vi "Project Open.vi"(8 "error in":errorcluster, 11 "File Path":path) -> (0 "error out":errorcluster caption="错误输出")   [LabVIEW 2016]
uses:
  DAQ-VirtualCH/SubVIs/VCH/Private/Ctrls/PSVCH_VCH Info.ctl
  DAQ-Config/SubVIs/FGV_Cards.ctl
  DAQ-Display/Controls/Global para Config.ctl
  DAQ-Config/Controls/PSCHN_Card Para.ctl
  DAQ-Config/Controls/PSCHN_Channel Para.ctl
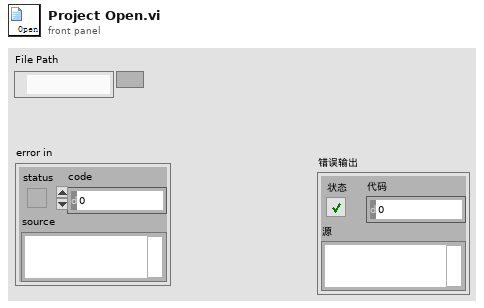
[diagram p1: front panel]
types:
  T1 = typedef "PSVCH_VCH Info.ctl" = cluster{"Tag":string[], "Tag String":string[], "Name":string[], "Enable":bool[], "Formula":string[], "Unit":string[], "Save":bool[], "Time":i64[]}
  T2 = typedef "Global para Config.ctl" = cluster{"连续存储设置":cluster{"Save Mode":i32, "Sel Save Mode":i32, "FolderPath":path, "Filename":string, "Explation":string, "AutoPoint":i32, "Template":path}, "Latest Prj":path, "Tdms Ref*":refnum<k34>, "默认波形图个数":u8, "列表列数":u8}
  T3 = typedef "PSCHN_Card Para.ctl" = cluster{"Module Type":string, "Module Name":string, "ModuSN":string, "ModuIP":string, "Used?":bool, "Connected":bool, "Timing*":cluster{"Sample Rate":dbl}, "Channels":T4[]}
  T4 = typedef "PSCHN_Channel Para.ctl" = cluster{"CHTag*":string, "Used?*":bool, "CHName":string, "Unit":string, "斜率":dbl, "截距":dbl}
  T5 = cluster{"DispXml[]":string[], "VCH Out":T1, "_Para":T2, "Cards":T3[], "CHTag[]":string[]}
  T6 = typedef "FGV_Cards.ctl" = enum16{"Initlize", "Set_DAQCards", "Set_VCHCards", "Get_DAQCards", "Get_VCHCards", "Get_ALLUsing"}
  T7 = enum16{"Run", "Pause", "Stop", "DAQ Chl", "Save", "Update Data", "Symbol Path", "DAQ DATA Queues", "None"}
  T8 = cluster{"Main Queue":string, "DAQ Queue":string, "ANA Queue":string, "CUI Queue":string, "Q-FocusList":string, "Q-Toolbar":string, "Q-Config":string}
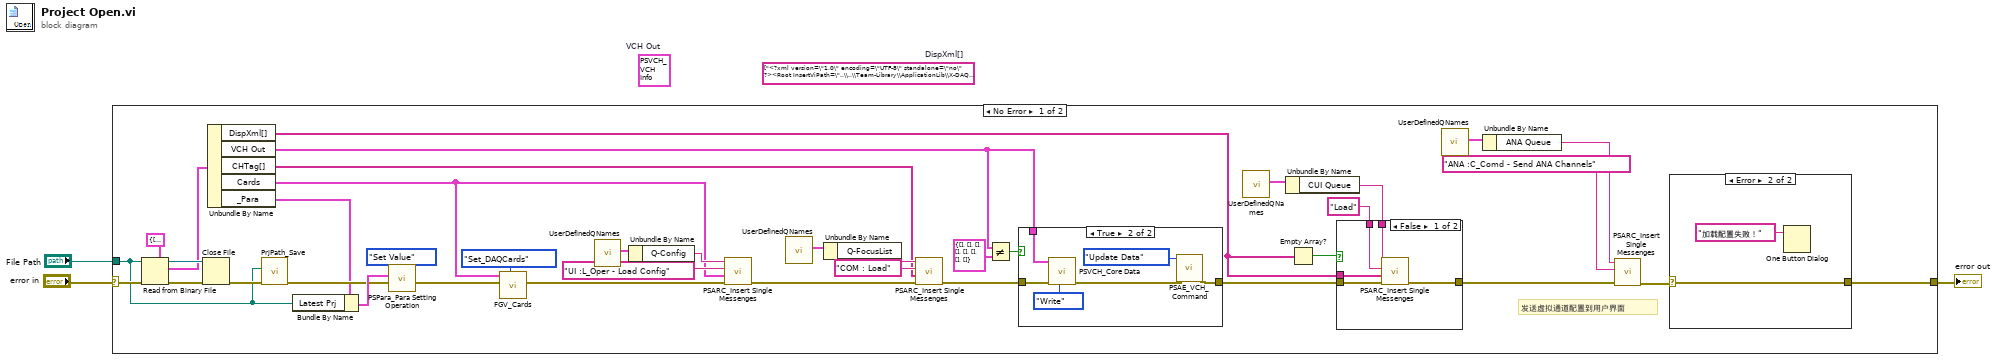
[diagram p0: block diagram]
diagram:
  (unwired) string[] ["<?xml version=\"1.0\" encoding=\"UTF-8\" standalone=\"no\" ?><Root InsertViPath=\"..\\..\\Team-Library\\ApplicationLib\\X-DAQ Viewer\\SubVIs\\New_GraphDispWithTime.vi\" InsertViValue=\"&lt;Cluster>\r&#xA;&lt;Name>ViValue&lt;/Name>\r&#xA;&lt;NumElts>5&lt;/NumElts>\r&#xA;&lt;String>\r&#xA;&lt;Name>CHTag&lt;/Name>\r&#xA;&lt;Val>&lt;/Val>\r&#xA;&lt;/String>\r&#xA;&lt;Cluster>\r&#xA;&lt;Name>GraphProperts&lt;/Name>\r&#xA;&lt;NumElts>3&lt;/NumElts>\r&#xA;&lt;DBL>\r&#xA;&lt;Name>YMax&lt;/Name>\r&#xA;&lt;Val>10.00000000000000&lt;/Val>\r&#xA;&lt;/DBL>\r&#xA;&lt;DBL>\r&#xA;&lt;Name>YMin&lt;/Name>\r&#xA;&lt;Val>0.00000000000000&lt;/Val>\r&#xA;&lt;/DBL>\r&#xA;&lt;U8>\r&#xA;&lt;Name>ScaleFit&lt;/Name>\r&#xA;&lt;Val>2&lt;/Val>\r&#xA;&lt;/U8>\r&#xA;&lt;/Cluster>\r&#xA;&lt;String>\r&#xA;&lt;Name>CHUnit&lt;/Name>\r&#xA;&lt;Val>&lt;/Val>\r&#xA;&lt;/String>\r&#xA;&lt;String>\r&#xA;&lt;Name>CHName&lt;/Name>\r&#xA;&lt;Val>&lt;/Val>\r&#xA;&lt;/String>\r&#xA;&lt;String>\r&#xA;&lt;Name>CHValue&lt;/Name>\r&#xA;&lt;Val>-----&lt;/Val>\r&#xA;&lt;/String>\r&#xA;&lt;/Cluster>\r&#xA;\" SplitMode=\"-1\"/>"]  # DispXml[]
  (unwired) T1 {"Tag"=["VCH1", "VCH2", "VCH3", "VCH4", "VCH5", "VCH6", "VCH7", "VCH8"], "Tag String"=["VCH1", "VCH2", "VCH3", "VCH4", "VCH5", "VCH6", "VCH7", "VCH8"], "Name"=["VCH1", "VCH2", "VCH3", "VCH4", "VCH5", "VCH6", "VCH7", "VCH8"], "Enable"=[FALSE, FALSE, FALSE, FALSE, FALSE, FALSE, FALSE, FALSE], "Formula"=["", "", "", "", "", "", "", ""], "Unit"=["V", "V", "V", "V", "V", "V", "V", "V"], "Save"=[TRUE, TRUE, TRUE, TRUE, TRUE, TRUE, TRUE, TRUE], "Time"=[1000, 1000, 1000, 1000, 1000, 1000, 1000, 1000]}  # VCH Out
  n1 = case shown="No Error" "error in" {
    selector: "error in" -> [w22 w59]
    tunnel: [w32 w59] -> w3
    tunnel: "File Path" -> [w20 _]
    frame No Error {
      # "发送虚拟通道配置到用户界面"
      n2 = Read from Binary File(5:T5 {"DispXml[]"=[], "VCH Out"={"Tag"=[], "Tag String"=[], "Name"=[], "Enable"=[], "Formula"=[], "Unit"=[], "Save"=[], "Time"=[]}, "_Para"={"连续存储设置"={"Save Mode"=0, "Sel Save Mode"=0, "FolderPath"=path "", "Filename"="", "Explation"="", "AutoPoint"=0, "Template"=path ""}, "Latest Prj"=path "", "Tdms Ref*"=refnum, "默认波形图个数"=0, "列表列数"=0}, "Cards"=[], "CHTag[]"=[]} ("输出簇"), 8:w22, 11:w20) -> (0:w41:errorcluster, 2:w17:T5, 3:w40:refnum<file>)  [unwired: 3 in, 1 out]
      n3 = Close File(refnum=w40, error in=w41) -> (error out=w21:errorcluster)  [unwired: 1 out]
      n4 = Unbundle By Name(w17) -> ("DispXml[]"=w16:string[], "VCH Out"=w15:T1, "CHTag[]"=w9:string[], "Cards"=w14:T3[], "_Para"=w5:T2)
      n5 = call "PrjPath_Save.vi"("error in (no error)"=w21, "Path"=w20) -> ("error out"=w7:errorcluster)  [unwired: 8 in]
      n6 = Bundle By Name(cluster=w5, "Latest Prj"=w20) -> (w31:T2)
      n7 = call "PSPara_Para Setting Operation.vi"("Operation"=enum16{"Set Value", "Get Value", "Initialize"}."Set Value", "error in (no error)"=w7, "_Para"=w31) -> ("error out"=w6:errorcluster)  [unwired: 7 in, 1 out]
      n8 = call "FGV_Cards.vi"("Action"=FGV_Cards."Set_DAQCards", "error in (no error)"=w6, "Cards in"=w14) -> ("error out"=w18:errorcluster)  [unwired: 7 in, 1 out]
      n9 = call "UserDefinedQNames.vi"() -> ("All Queues"=w24:T8)  [unwired: 11 in]
      n10 = Unbundle By Name(w24) -> ("Q-Config"=w23:string)
      n11 = call <vilib>:"PSARC_Insert Single Messenges.vi"("error in (no error)"=w18, "Data"=w14, "Order"="UI :L_Oper - Load Config", "Queue Name"=w23) -> ("error out"=w10:errorcluster)  [unwired: 7 in]
      n12 = call "UserDefinedQNames.vi"() -> ("All Queues"=w13:T8)  [unwired: 11 in]
      n13 = Unbundle By Name(w13) -> ("Q-FocusList"=w12:string)
      n14 = call <vilib>:"PSARC_Insert Single Messenges.vi"("error in (no error)"=w10, "Data"=w9, "Order"="COM : Load", "Queue Name"=w12) -> ("error out"=w8:errorcluster)  [unwired: 7 in]
      n15 = Not Equal?(x=w15, y=T1 {"Tag"=[], "Tag String"=[], "Name"=[], "Enable"=[], "Formula"=[], "Unit"=[], "Save"=[], "Time"=[]}) -> (x != y?=w29:bool)
      n16 = case shown="True" w29 {
        tunnel: w8 -> [w49 w54]
        tunnel: [w49 w51] -> w37
        tunnel: w15 -> [_ w50]
        frame False {
        }
        frame True {
          n17 = call "PSVCH_Core Data.vi"("Oper"=enum16{"Init", "Read", "Write"}."Write", "Error In (no error)"=w54, "VCH In"=w50) -> ("Error Out"=w52:errorcluster)  [unwired: 7 in, 1 out]
          n18 = call "PSAE_VCH_Command.vi"("Error In (no error)"=w52, "Comd"=T7."Update Data") -> ("Error Out"=w51:errorcluster)  [unwired: 9 in]
        }
      }
      n19 = call "UserDefinedQNames.vi"() -> ("All Queues"=w26:T8)  [unwired: 11 in]
      n20 = Unbundle By Name(w26) -> ("CUI Queue"=w25:string)
      n21 = Empty Array?(array=w16) -> (empty?=w28:bool)
      n22 = case shown="False" w28 {
        tunnel: w25 -> [w47 _]
        tunnel: "Load" ("Queue Name(unamed)") -> [w46 _]
        tunnel: w37 -> [w45 w48]
        tunnel: [w44 w48] -> w36
        tunnel: w16 -> [w43 _]
        frame False {
          n23 = call <vilib>:"PSARC_Insert Single Messenges.vi"("error in (no error)"=w45, "Data"=w43, "Order"=w46, "Queue Name"=w47) -> ("error out"=w44:errorcluster)  [unwired: 7 in]
        }
        frame True {
        }
      }
      n24 = call "UserDefinedQNames.vi"() -> ("All Queues"=w27:T8)  [unwired: 11 in]
      n25 = Unbundle By Name(w27) -> ("ANA Queue"=w34:string)
      n26 = call <vilib>:"PSARC_Insert Single Messenges.vi"("error in (no error)"=w36, "Order"="ANA :C_Comd - Send ANA Channels", "Queue Name"=w34) -> ("error out"=w33:errorcluster)  [unwired: 8 in]
      n27 = case shown="Error" w33 {
        selector: w33 -> [w56 w58]
        tunnel: [w56 w58] -> w32
        frame No Error {
        }
        frame Error {
          n28 = One Button Dialog(message="加载配置失败！" ("消息")) -> ()  [unwired: 1 in, 1 out]
        }
      }
    }
    frame Error {
    }
  }
  "error out" <- w3
